vi "validateMonochromatorRanges.vi"(6 "wavelength":T2=400.0, 8 "error in (no error)":errorcluster, 9 "Exit Slit Width":T1, 10 "Entrance Slit Width":T1, 11 "MonoClientCommunicator in":refnum<class "MonoClientCommunicator.lvclass">) -> (0 "error out":errorcluster, 1 "exsInRange":bool, 2 "ensInRange":bool, 3 "MonoClientCommunicator out":refnum<class "MonoClientCommunicator.lvclass">, 4 "wavelengthInRange":bool, 5 "gratingInRange":bool)   [LabVIEW 2016, in "MonoClientCommunicator.lvclass"]
uses:
  MonoClientCommunicator.lvclass
  Typedefs/slitWidth.ctl
  Typedefs/wavelength.ctl
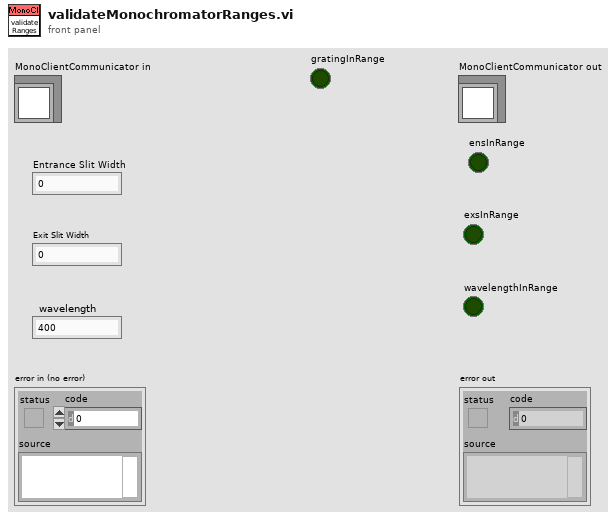
[diagram p1: front panel]
types:
  T1 = typedef "slitWidth.ctl" = dbl
  T2 = typedef "wavelength.ctl" = dbl
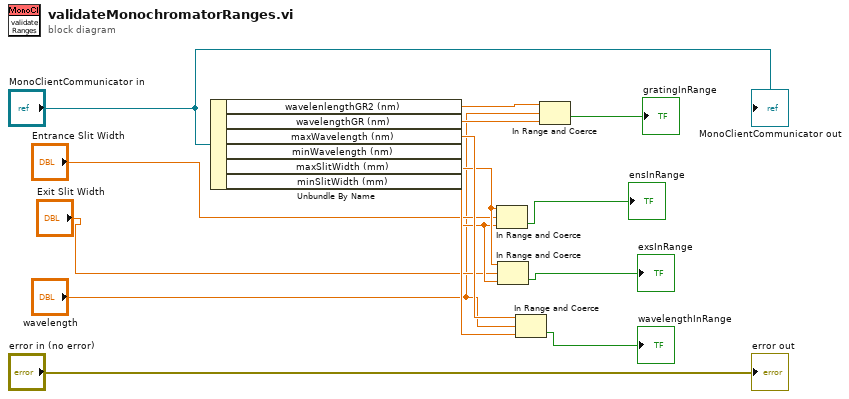
[diagram p0: block diagram]
diagram:
  n1 = Unbundle By Name("MonoClientCommunicator in") -> ("wavelenlengthGR2 (nm)"=w4:sgl, "wavelengthGR (nm)"=w3:sgl, "maxWavelength (nm)"=w13:sgl, "minWavelength (nm)"=w12:sgl, "maxSlitWidth (mm)"=w11:sgl, "minSlitWidth (mm)"=w10:sgl)
  n2 = In Range and Coerce(upper limit=w11, x="Entrance Slit Width", lower limit=w10) -> (In Range?=→"ensInRange":bool)  [unwired: 1 out]
  n3 = In Range and Coerce(upper limit=w11, x="Exit Slit Width", lower limit=w10) -> (In Range?=→"exsInRange":bool)  [unwired: 1 out]
  n4 = In Range and Coerce(upper limit=w13, x="wavelength", lower limit=w12) -> (In Range?=→"wavelengthInRange":bool)  [unwired: 1 out]
  n5 = In Range and Coerce(upper limit=w4, x="wavelength", lower limit=w3) -> (In Range?=→"gratingInRange":bool)  [unwired: 1 out]
  "error out" <- "error in (no error)"
  "MonoClientCommunicator out" <- "MonoClientCommunicator in"
